vi "Untitled 1.vi"   [LabVIEW 2015]
uses:
  <vilib>/rvi/Emulation/niFpgaGetClockAttributes.vi
  <vilib>/rvi/Emulation/niFpgaSctlEmulationGetInTimedLoop.vi
  <vilib>/rvi/Emulation/niFpgaEmulationReportErrorSimple.vi
  <vilib>/rvi/eio/common/nirviEmuTemplateMethod_errors.vi
  <vilib>/rvi/Emulation/niFpgaCriticalErrorInLSC.vi
  <vilib>/eio/EIONode/EIONode.xnode
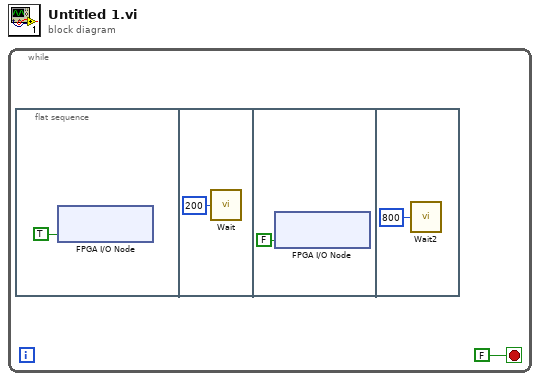
[diagram p0: block diagram]
diagram:
  n1 = while {
    stop <- FALSE stop-if-true
    n2 = flat-sequence {
      frame #0 {
        n3 = xnode "FPGA I/O Node"("FPGA LED"=TRUE) -> ()  [unwired: 1 in, 1 out]
      }
      frame #1 {
        n4 = call "Wait"("Count(mSec)"=u32 200) -> ()  [unwired: 1 out]
      }
      frame #2 {
        n5 = xnode "FPGA I/O Node"("FPGA LED"=FALSE) -> ()  [unwired: 1 in, 1 out]
      }
      frame #3 {
        n6 = call "Wait2"("Count(mSec)"=u32 800) -> ()  [unwired: 1 out]
      }
    }
  }
